vi "CMD_ABS_POS.vi"(9 "Chan Ident":string="1", 10 "absolute position/mm":i32=10) -> (1 "Command":string)   [LabVIEW 2017]
panel:
  out "concatenated string":string
  out "x = y?":bool
  in  "ReqCmd 2":string="\u0004d040600A2010100400D0300"
  # "CMD_ABS_POS"
  # "TX 53, 04, 06, 00, A2, 01, 01, 00, 40, 0D, 03, 00,"
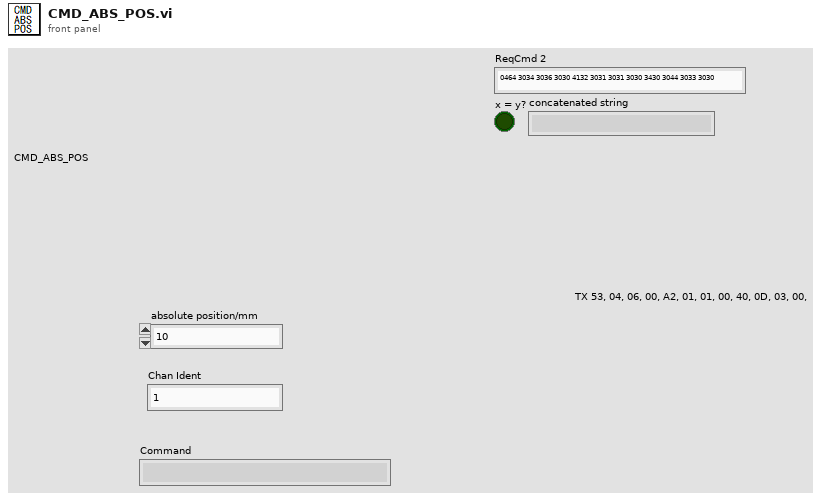
[diagram p1: front panel]
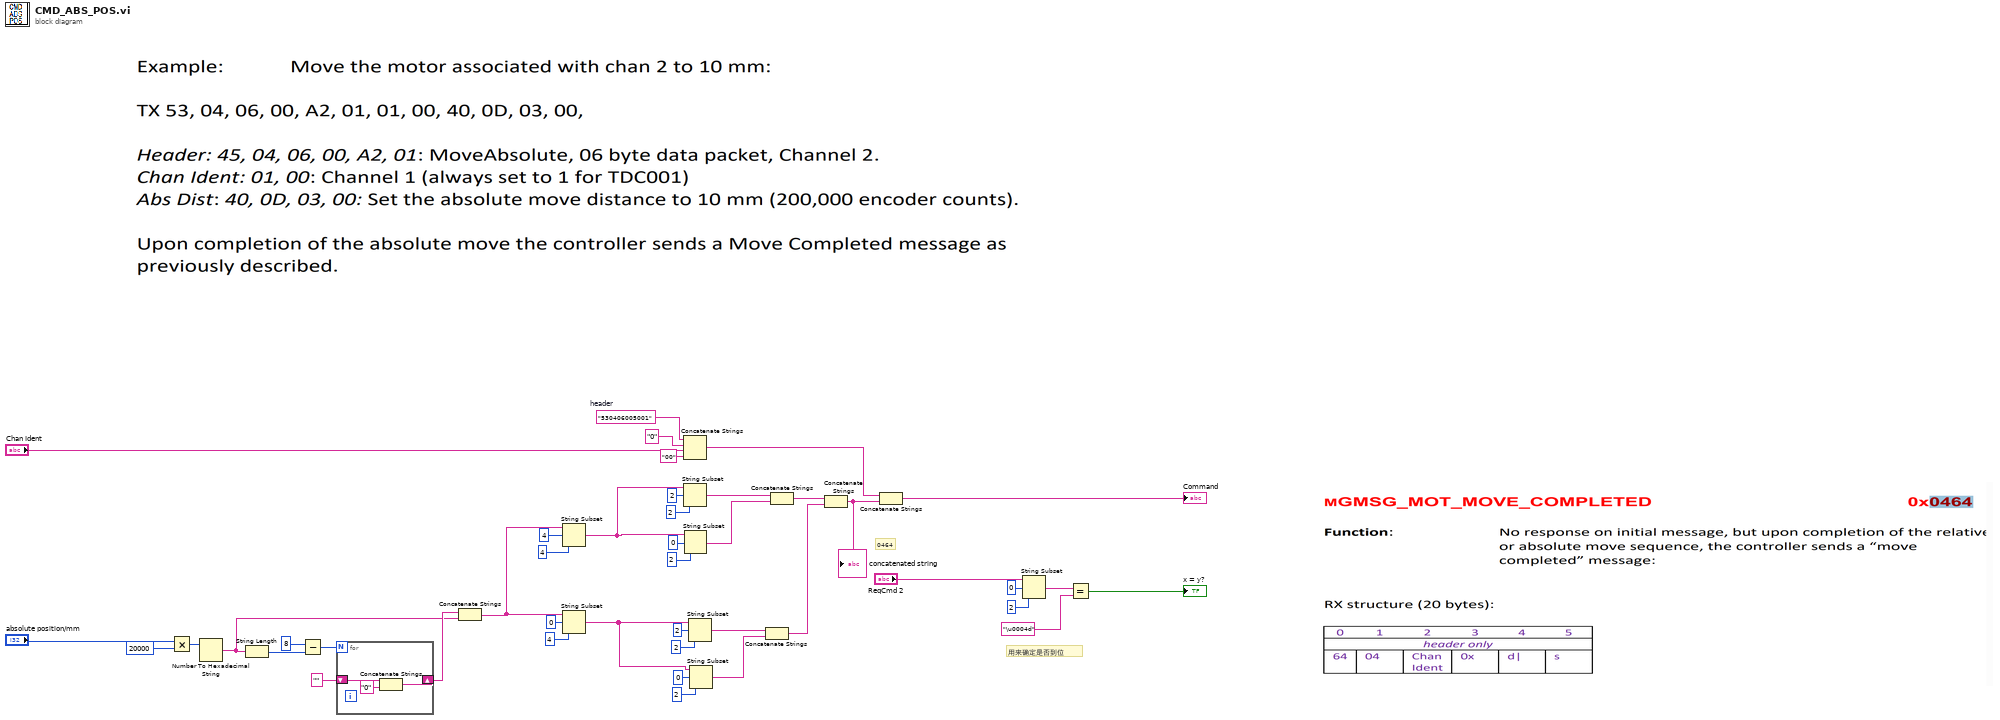
[diagram p0: block diagram]
diagram:
  w10 = "530406005001"  # header
  # "用来确定是否到位"
  # "0464"
  n1 = Multiply(x="absolute position/mm", y=20000) -> (x*y=w36:i32)
  n2 = Number To Hexadecimal String(2:w36) -> (0:w30:string)  [unwired: 1 in]
  n3 = String Length(string=w30) -> (length=w42:i32)
  n4 = Subtract(x=8, y=w42) -> (x-y=w41:i32)
  n5 = for {
    N: w41 -> [_]
    shift-right: [w44] -> w39
    shift-left: "" -> [w46]
    n6 = Concatenate Strings(w46, "0" ("字符串")) -> (w44:string)
  }
  n7 = Concatenate Strings(w39, w30) -> (w31:string)
  n8 = String Subset(string=w31, offset (0)=4 ("偏移量(0)"), length (rest)=4 ("长度（剩余）")) -> (substring=w25:string)
  n9 = String Subset(string=w31, offset (0)=0 ("偏移量(0)"), length (rest)=4 ("长度（剩余）")) -> (substring=w18:string)
  n10 = Concatenate Strings(w10, "0" ("字符串"), "Chan Ident", "00" ("string")) -> (w9:string)
  n11 = String Subset(string=w25, offset (0)=2 ("偏移量(0)"), length (rest)=2 ("长度（剩余）")) -> (substring=w24:string)
  n12 = String Subset(string=w25, offset (0)=0 ("偏移量(0)"), length (rest)=2 ("长度（剩余）")) -> (substring=w23:string)
  n13 = String Subset(string=w18, offset (0)=2 ("偏移量(0)"), length (rest)=2 ("长度（剩余）")) -> (substring=w17:string)
  n14 = String Subset(string=w18, offset (0)=0 ("偏移量(0)"), length (rest)=2 ("长度（剩余）")) -> (substring=w16:string)
  n15 = Concatenate Strings(w17, w16) -> (w14:string)
  n16 = Concatenate Strings(w24, w23) -> (w15:string)
  n17 = Concatenate Strings(w15, w14) -> (w13:string)
  "concatenated string" <- w13
  n18 = Concatenate Strings(w9, w13) -> (→"Command":string)
  n19 = String Subset(string="ReqCmd 2", offset (0)=0 ("偏移量(0)"), length (rest)=2 ("长度（剩余）")) -> (substring=w4:string)
  n20 = Equal?(x=w4, y="\u0004d") -> (x = y?=→"x = y?":bool)
